vi "HeaterRead.vi"(8 "Error In":errorcluster) -> (0 "Error Out":errorcluster)   [LabVIEW 2012]
uses:
  HeaterConfigurationGlobalAction.ctl
  libs/Omega-CSi32/Omega-CSi32.lvlib
  libs/LV-Utilities/LV-Utilities.lvlib
panel:
  out "Temperature":dbl[](array[numeric])
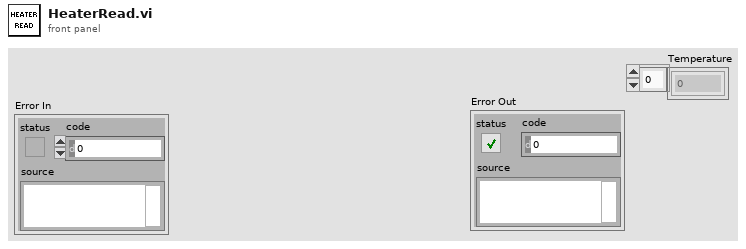
[diagram p1: front panel]
types:
  T1 = typedef "HeaterConfigurationGlobalAction.ctl" = enum16{"Init", "Get", "Set", "Add", "Remove", "Reset"}
  T2 = typedef "HeaterConfiguration.ctl" = cluster{"VISA Resource":refnum<visa-resource-name>, "COM Port":u8, "Setpoint":dbl, "Standby?":bool}
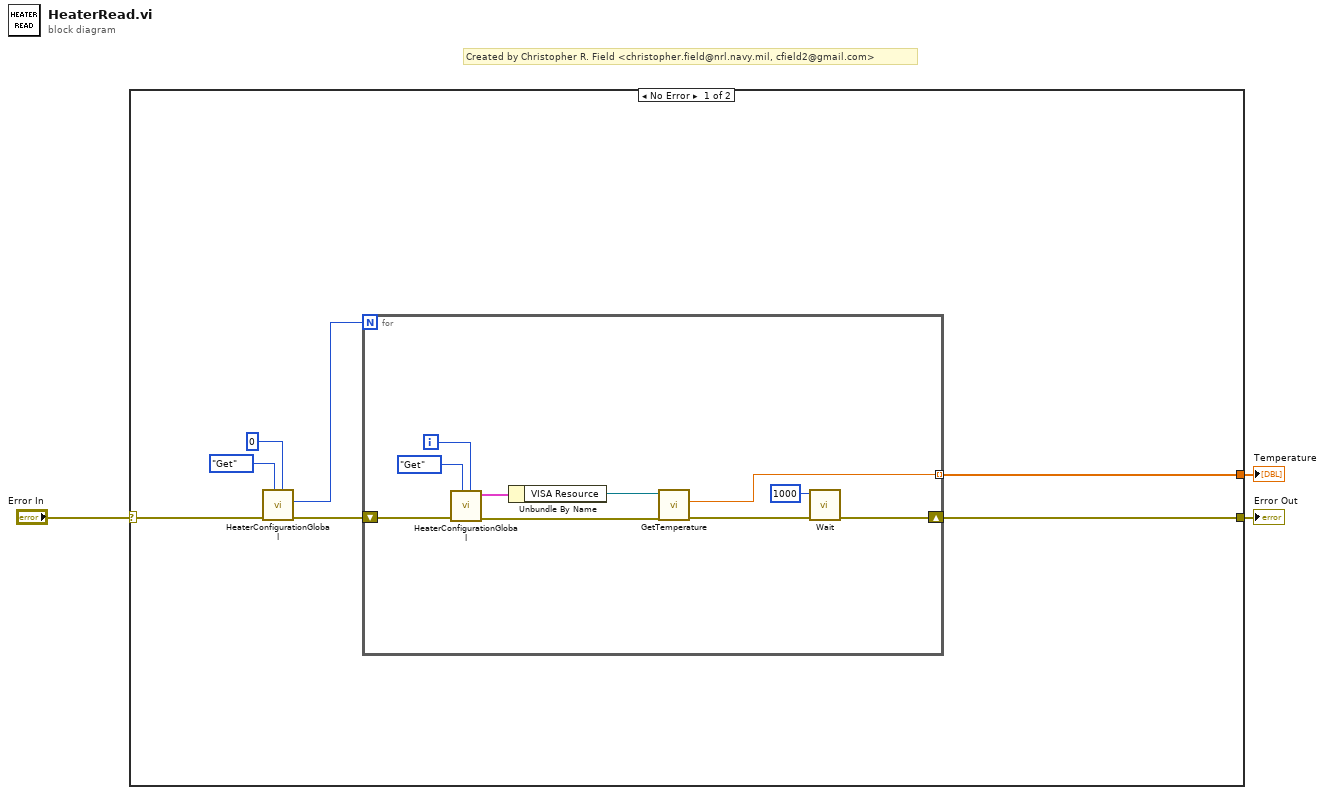
[diagram p0: block diagram]
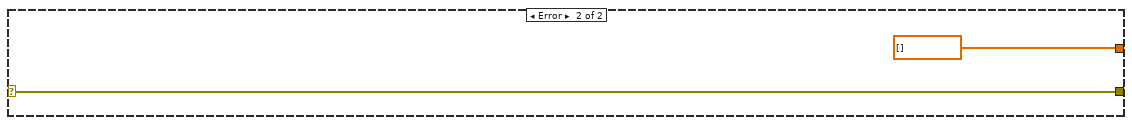
[diagram p2: hidden frame]
diagram:
  # "Created by Christopher R. Field <christopher.field@nrl.navy.mil, cfield2@gmail.com>"
  n1 = case shown="No Error" "Error In" {
    selector: "Error In" -> [w5 w22]
    tunnel: [w10 w22] -> w1
    tunnel: [w9 dbl[] []] -> w2
    frame No Error {
      n2 = call "HeaterConfigurationGlobal.vi"("Index"=u16 0, "Action"=HeaterConfigurationGlobalAction."Get", "Error In"=w5) -> ("Error Out"=w4:errorcluster, "Heater Count"=w8:i32)  [unwired: 6 in, 1 out]
      n3 = for {
        N: w8 -> [_]
        tunnel: [w17] -> w9 mode=indexing
        shift-right: [w18] -> w10
        shift-left: w4 -> [w11]
        i -> [w16]
        n4 = call "HeaterConfigurationGlobal.vi"("Index"=w16, "Action"=HeaterConfigurationGlobalAction."Get", "Error In"=w11) -> ("Error Out"=w12:errorcluster, "Value Out"=w14:T2)  [unwired: 6 in, 1 out]
        n5 = Unbundle By Name(w14) -> ("VISA Resource"=w13:refnum<visa-resource-name>)
        n6 = call "GetTemperature.vi"("Error In"=w12, "Omega CSi32 In"=w13) -> ("Error Out"=w20:errorcluster, "Temperature (C)"=w17:dbl)  [unwired: 6 in, 2 out]
        n7 = call "Wait.vi"("Error In"=w20, "Wait Time (msec)"=u32 1000) -> ("Error Out"=w18:errorcluster)  [unwired: 9 in]
      }
    }
    frame Error {
    }
  }
  "Error Out" <- w1
  "Temperature" <- w2
